vi "Read.vi"(8 "error in (no error)":errorcluster, 11 "VISA resource name":refnum<visa-resource-name>) -> (0 "error out":errorcluster, 1 "Secondary Parameter":dbl, 2 "Primary Parameter":dbl, 3 "VISA resource name out":refnum<visa-resource-name>)   [LabVIEW 2017, in "Agilent E4980.lvlib"]
doc: "Takes measurements from the instrument."
uses:
  Agilent E4980.lvlib
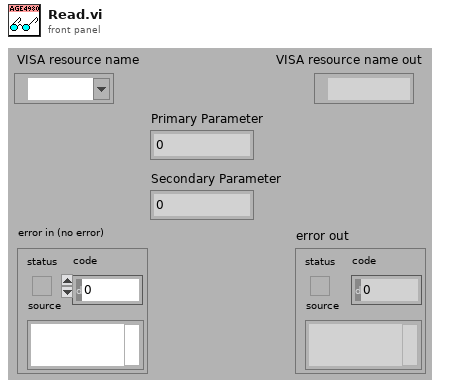
[diagram p1: front panel]
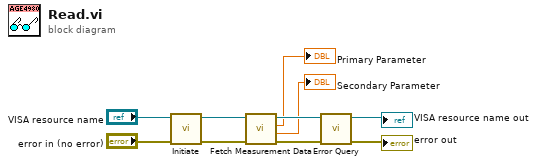
[diagram p0: block diagram]
diagram:
  n1 = call "Initiate.vi"("error in (no error)"="error in (no error)", "VISA resource name"="VISA resource name") -> ("error out"=w7:errorcluster, "VISA resource name out"=w8:refnum<visa-resource-name>)  [unwired: 8 in]
  n2 = call "Fetch Measurement Data.vi"("error in (no error)"=w7, "VISA resource name"=w8) -> ("error out"=w5:errorcluster, "Secondary Parameter"=→"Secondary Parameter":dbl, "Primary Parameter"=→"Primary Parameter":dbl, "VISA resource name out"=w6:refnum<visa-resource-name>)  [unwired: 5 in, 1 out]
  n3 = call "Error Query.vi"("error in (no error)"=w5, "VISA resource name"=w6) -> ("error out"=→"error out":errorcluster, "VISA resource name out"=→"VISA resource name out":refnum<visa-resource-name>)  [unwired: 6 in, 2 out]
